vi "read_qr.vi"(7 "error in":errorcluster) -> (0 "error out":errorcluster, 2 "Data":string)   [LabVIEW 2018]
uses:
  <vilib>/vision/Instrument.llb/QR Code Search Options.ctl
  <vilib>/vision/Instrument.llb/Demodulation Mode.ctl
  <vilib>/vision/Instrument.llb/Cell Sample Size.ctl
  <vilib>/vision/Instrument.llb/Cell Filter Mode.ctl
  <vilib>/vision/Instrument.llb/QR Code Description Options.ctl
  <vilib>/vision/Instrument.llb/Data Matrix Polarity.ctl
  <vilib>/vision/Instrument.llb/QR Code Model Type.ctl
  <vilib>/vision/NI_Vision_Development_Module.lvlib
panel:
  out "Found?":bool
  in  "qr_image":bool
  in  "QR Description Options":T1={"Matrix Size (cells)"=0, "Barcode Polarity"=-2, "Mirror Mode"=-2, "QR Model"=0} {"Mirror Mode" items=["Auto-detect"=-2, "Normal"=0, "Mirrored"=1]; "Matrix Size (cells)" items=["Auto-detect"=0, "11x11 - Version 1 (Micro QR Only)"=11, "13x13 - Version 2 (Micro QR Only)"=13, "15x15 - Version 3 (Micro QR Only)"=15, "17x17 - Version 4 (Micro QR Only)"=17, "21x21 - Version 1"=21, "25x25 - Version 2"=25, "29x29 - Version 3"=29, "33x33 - Version 4"=33, "37x37 - Version 5"=37, "41x41 - Version 6"=41, "45x45 - Version 7"=45, "49x49 - Version 8"=49, "53x53 - Version 9"=53, "57x57 - Version 10"=57, "61x61 - Version 11"=61, "65x65 - Version 12"=65, "69x69 - Version 13"=69, "73x73 - Version 14"=73, "77x77 - Version 15"=77, "81x81 - Version 16"=81, "85x85 - Version 17"=85, "89x89 - Version 18"=89, "93x93 - Version 19"=93, "97x97 - Version 20"=97, "101x101 - Version 21"=101, "105x105 - Version 22"=105, "109x109 - Version 23"=109, "113x113 - Version 24"=113, "117x117 - Version 25"=117, "121x121 - Version 26"=121, "125x125 - Version 27"=125, "129x129 - Version 28"=129, "133x133 - Version 29"=133, "137x137 - Version 30"=137, "141x141 - Version 31"=141, "145x145 - Version 32"=145, "149x149 - Version 33"=149, "153x153 - Version 34"=153, "157x157 - Version 35"=157, "161x161 - Version 36"=161, "165x165 - Version 37"=165, "169x169 -  Version 38"=169, "173x173 - Version 39"=173, "177x177 - Version 40"=177]; "QR Model" items=["Auto-detect", "Micro", "Model 1", "Model 2"]; "Barcode Polarity" items=["Auto-detect"=-2, "Black on White"=0, "White on Black"=1]}
  in  "ROI Descriptor":T4 {"Contours"."Type" items=["No Selection", "Point", "Line", "Rectangle", "Oval", "Polygon", "Freehand Region", "Annulus", "Unused2", "Unused3", "Broken Line", "Freehand Line", "Rotated Rectangle"]}
  in  "QR Search Options":T5={"Rotation Mode"=enum."Unlimited", "Skip Location?"=FALSE, "Edge Threshold"=30, "Demodulation Mode"=-2, "Cell Sample Size"=-2, "Cell Filter Mode"=-2, "Skew Degrees Allowed"=5} {"Cell Filter Mode" items=["Auto-detect"=-2, "Average"=0, "Median"=1, "Central Average"=2, "High Average"=3, "Low Average"=4, "Very High Average"=5, "Very Low Average"=6, "All Filters"=8]; "Cell Sample Size" items=["Auto-detect"=-2, "1x1"=1, "2x2"=2, "3x3"=3, "4x4"=4, "5x5"=5, "6x6"=6, "7x7"=7]; "Demodulation Mode" items=["Auto-detect"=-2, "Histogram"=0, "Local Contrast"=1, "Combination"=2, "All"=3]}
  out "Image Out":T9(plugin-control)
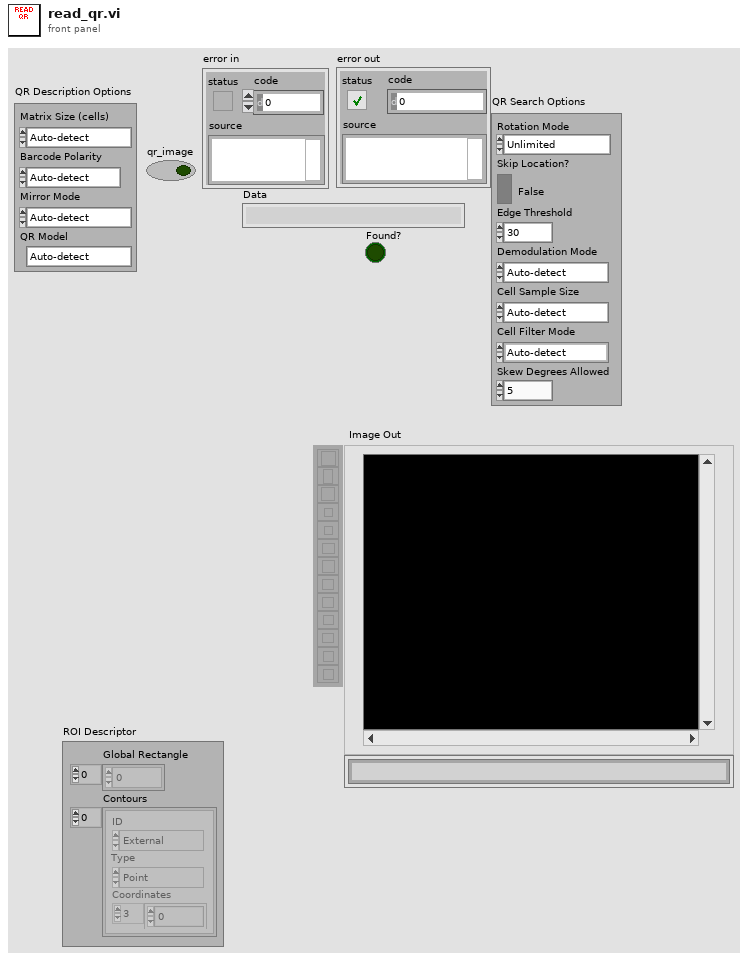
[diagram p1: front panel]
types:
  T1 = typedef "QR Code Description Options.ctl" = cluster{"Matrix Size (cells)":i32, "Barcode Polarity":T2, "Mirror Mode":i32, "QR Model":T3}
  T2 = typedef "Data Matrix Polarity.ctl" = i32
  T3 = typedef "QR Code Model Type.ctl" = i32
  T4 = typedef "ROI Descriptor" = cluster{"Global Rectangle":i32[], "Contours":cluster{"ID":enum32{"External", "Internal"}, "Type":u32, "Coordinates":i32[]}[]}
  T5 = typedef "QR Code Search Options.ctl" = cluster{"Rotation Mode":enum32{"Unlimited", "0 Degrees", "90 Degrees", "180 Degrees", "270 Degrees"}, "Skip Location?":bool, "Edge Threshold":u32, "Demodulation Mode":T6, "Cell Sample Size":T7, "Cell Filter Mode":T8, "Skew Degrees Allowed":u32}
  T6 = typedef "Demodulation Mode.ctl" = i32
  T7 = typedef "Cell Sample Size.ctl" = i32
  T8 = typedef "Cell Filter Mode.ctl" = i32
  T9 = typedef "IMAQ Image.ctl" = refnum<image>
  T10 = typedef "QR Code Report.ctl" = cluster{"Found?":bool, "Data":string, "Bounding Box":cluster{"x":sgl, "y":sgl}[], "Errors Corrected":u32, "Dimensions (Rows/Cols)":u32, "Version":u32, "QR Model":T3, "Stream Mode":T11, "Barcode Polarity":T2, "Mirrored?":bool, "Append Stream Position":u32, "Size of Append Stream":u32, "First EAN-128 ID":i32, "First Alternate Language ID":i32, "Append Stream ID":u32, "Minimum Edge Strength":u32, "Demodulation Mode":T6, "Cell Sample Size":T7, "Cell Filter Mode":T8}
  T11 = typedef "QR Code Stream Mode Type.ctl" = i32
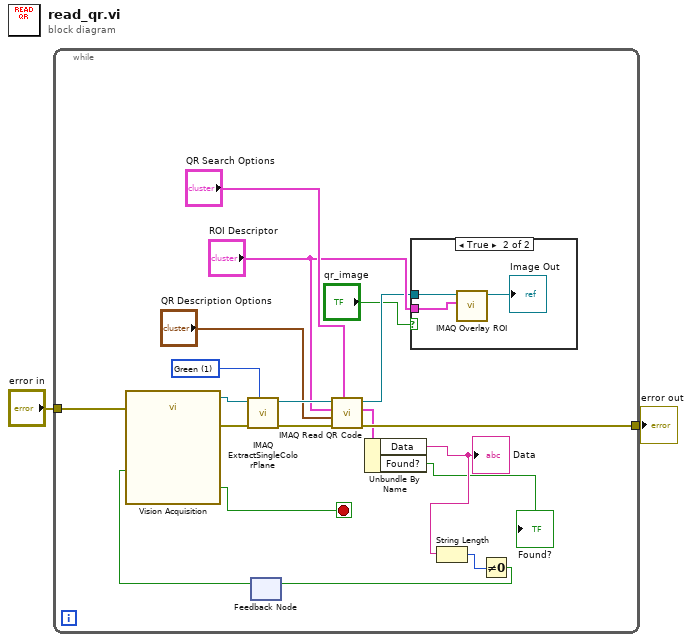
[diagram p0: block diagram]
diagram:
  n1 = while {
    tunnel: [w17] -> w1
    tunnel: "error in" -> [w10]
    stop <- w8 stop-if-true
    w18 = 1 items=["Red", "Green", "Blue", "Hue", "Saturation", "Luminance", "Value", "Intensity"] ("Color Plane")
    n2 = feedback #1() -> (w4:bool)  [unwired: 1 in]
    n3 = call "Vision Acquisition"("Stop (F)"=w4, "error in"=w10) -> ("Image Out"=w16:T9, "Stopped"=w8:bool, "error out"=w15:errorcluster)  [unwired: 22 in, 1 out]
    n4 = call "IMAQ ExtractSingleColorPlane"("Color Plane"=w18, "error in (no error)"=w15, "Image Src"=w16) -> ("error out"=w20:errorcluster, "Image Dst Out"=w19:T9)  [unwired: 7 in]
    n5 = call "IMAQ Read QR Code"("QR Search Options"="QR Search Options", "error in (no error)"=w20, "QR Description Options"="QR Description Options", "ROI Descriptor"="ROI Descriptor", "Image"=w19) -> ("error out"=w17:errorcluster, "QR Code Report"=w9:T10, "Image (duplicate)"=w12:T9)  [unwired: 3 in, 1 out]
    n6 = Unbundle By Name(w9) -> ("Data"=w7:string, "Found?"=→"Found?":bool)
    "Data" <- w7
    n7 = case shown="True" "qr_image" {
      tunnel: "ROI Descriptor" -> [_ w23]
      tunnel: w12 -> [_ w22]
      frame False {
      }
      frame True {
        n8 = call "IMAQ Overlay ROI"("ROI Descriptor"=w23, "Image"=w22) -> ("Image Out"=→"Image Out":T9)  [unwired: 8 in, 1 out]
      }
    }
    n9 = String Length(string=w7) -> (length=w6:i32)
    n10 = Not Equal To 0?(x=w6) -> (x != 0?=w5:bool)
    n11 = feedback-in #1(w5) -> ()
  }
  "error out" <- w1
